vi "DIO Bit Write_Array.vi"(0 "DIO Device":tag, 5 "Port":string, 7 "data":bool[](array[boolean])=[TRUE, TRUE, TRUE, TRUE, TRUE, TRUE, TRUE, TRUE], 11 "error in (no error)":errorcluster) -> (15 "error out":errorcluster)   [LabVIEW 2022 SP3, in "niMIO.lvclass"]
uses:
  niMIO.lvclass
  <vilib>/DAQmx/write.llb/DAQmx Write (Digital 1D Bool 1Chan 1Samp).vi
  <vilib>/DAQmx/create/channels.llb/DAQmx Create Channel (DO-Digital Output).vi
  <vilib>/DAQmx/miscellaneous.llb/DAQmx Fill In Error Info.vi
  niMIO.lvclass/niMIO.ctl
panel:
  out "niDIO out":refnum<class "niMIO.lvclass">
  in  "niDIO in":refnum<class "niMIO.lvclass">
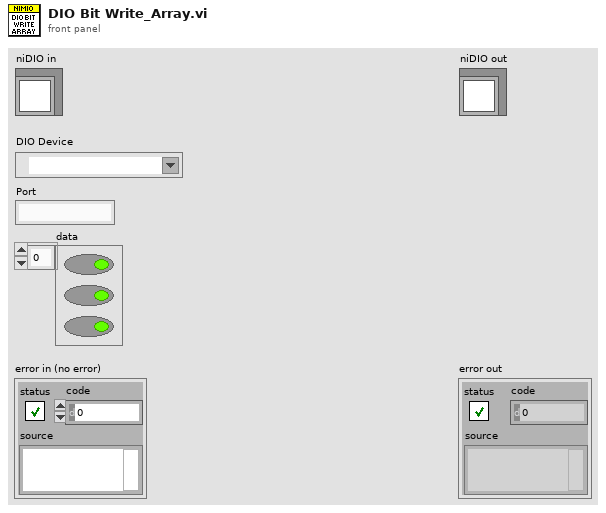
[diagram p1: front panel]
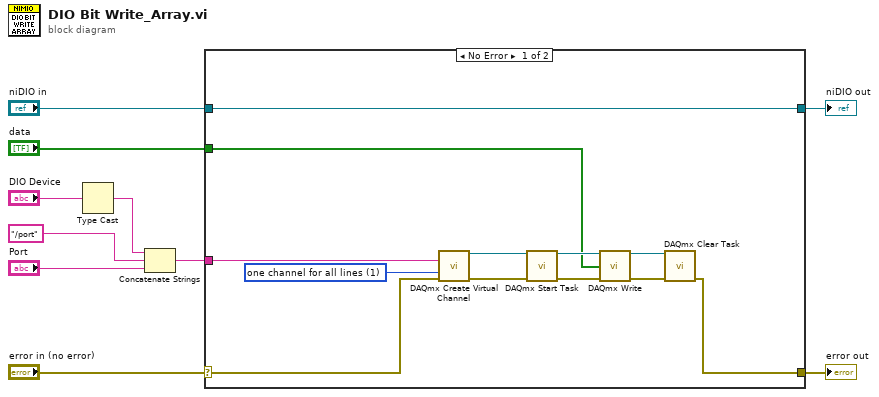
[diagram p0: block diagram]
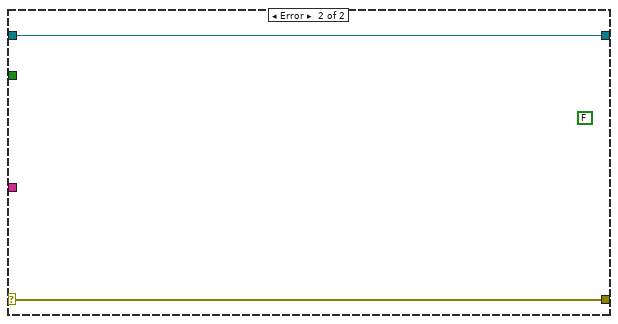
[diagram p2: hidden frame]
diagram:
  n1 = Type Cast(x="DIO Device") -> (*(type *) &x=w4:string)  [unwired: 1 in]
  n2 = Concatenate Strings(w4, "/port", "Port") -> (w2:string)
  n3 = case shown="No Error" "error in (no error)" {
    selector: "error in (no error)" -> [w13 w24]
    tunnel: [w12 w24] -> w9
    tunnel: [w22 w23] -> w7
    tunnel: "niDIO in" -> [w22 w23]
    tunnel: w2 -> [w14 _]
    tunnel: "data" -> [w11 _]
    frame No Error {
      w19 = 1 items=["one channel for each line", "one channel for all lines"] ("line grouping")
      n4 = call-poly <vilib>:"DAQmx Create Virtual Channel.vi"("lines"=w14, "line grouping"=w19, "error in"=w13) -> ("task out"=w21:refnum<k21>, "error out"=w20:errorcluster)  [unwired: 11 in]
      n5 = call <vilib>:"DAQmx Start Task.vi"("task/channels in"=w21, "error in"=w20) -> ("task out"=w18:refnum<k21>, "error out"=w17:errorcluster)  [unwired: 12 in]
      n6 = call-poly <vilib>:"DAQmx Write.vi"("task/channels in"=w18, "data"=w11, "error in"=w17) -> ("task out"=w16:refnum<k21>, "error out"=w15:errorcluster)  [unwired: 10 in, 1 out]
      n7 = call <vilib>:"DAQmx Clear Task.vi"("task in"=w16, "error in"=w15) -> ("error out"=w12:errorcluster)  [unwired: 13 in]
    }
    frame Error {
      (unwired) FALSE ("data")
    }
  }
  "error out" <- w9
  "niDIO out" <- w7
